vi "Extract_Country_List.vi"(5 "Raw Data Array (String)":string[][](array[string])) -> (0 "List of Countries":string[](array[string]), 2 "Raw Data Array Out (String)":string[][](array[string]))   [LabVIEW 2015]
doc: "This VI extracts the countries listed in the csv file to populate the drop-down menu"
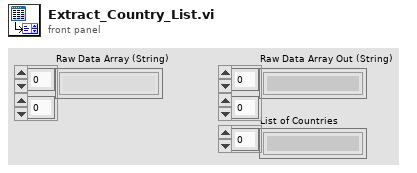
[diagram p1: front panel]
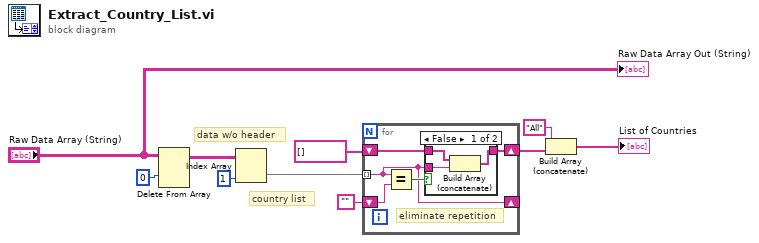
[diagram p0: block diagram]
diagram:
  # "country list"
  # "data w/o header"
  n1 = Delete From Array(array="Raw Data Array (String)", index (row)=0) -> (array with subset deleted=w3:string[][])  [unwired: 2 in, 1 out]
  n2 = Index Array(array=w3, index (col)=1 ("index (row)")) -> (element=w2:string[])  [unwired: 1 in]
  n3 = for {
    tunnel: w2 -> [w11] mode=indexing
    shift-right: [w11] -> _
    shift-left: "" -> [w15]
    shift-right: [w13] -> w8
    shift-left: string[] [] -> [w14]
    # "eliminate repetition"
    n4 = Equal?(x=w11, y=w15) -> (x = y?=w12:bool)
    n5 = case shown="False" w12 {
      tunnel: w14 -> [w18 w19]
      tunnel: [w17 w19] -> w13
      tunnel: w11 -> [w16 _]
      frame False {
        n6 = Build Array (concatenate)(w18, w16) -> (w17:string[])
      }
      frame True {
      }
    }
  }
  n7 = Build Array (concatenate)("All", w8) -> (→"List of Countries":string[])
  "Raw Data Array Out (String)" <- "Raw Data Array (String)"
